vi "Eredmények FIFO-ba.vi"(8 "error in (no error)":errorcluster, 11 "Analog data":T1) -> (0 "error out":errorcluster, 3 "Analog data out":T1)   [LabVIEW 2014]
uses:
  Analog data.ctl
panel:
  out "Waveform Graph":dbl[](graph)
  out "Resistance":dbl
  out "Temperature":dbl
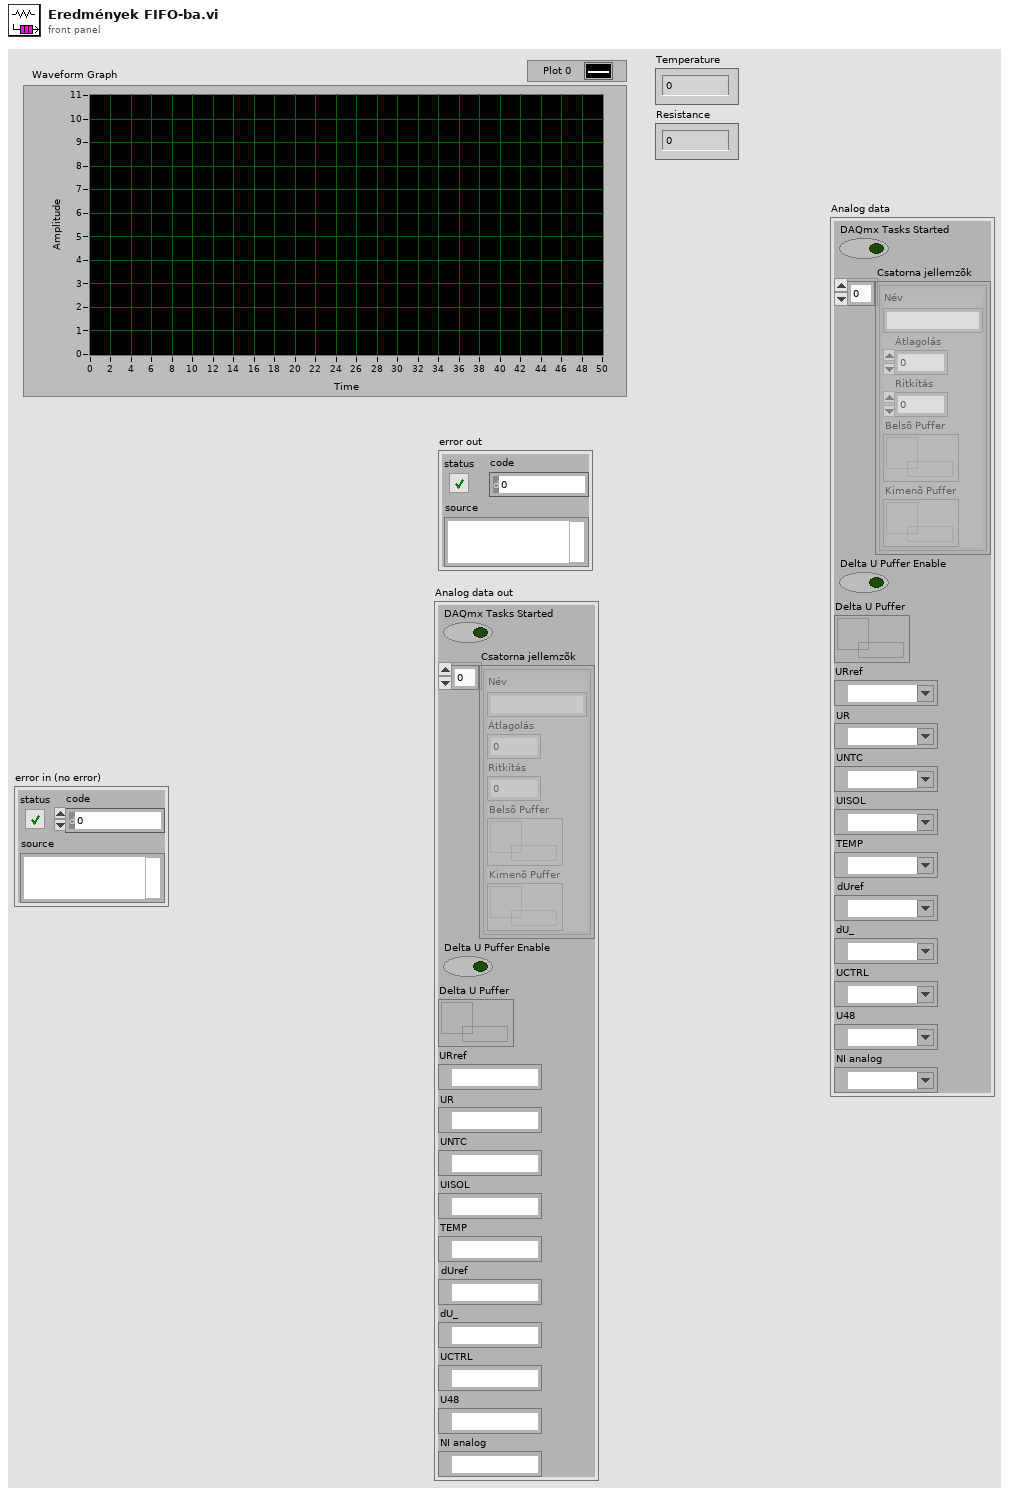
[diagram p1: front panel]
types:
  T1 = typedef "Analog data.ctl" = cluster{"DAQmx Tasks Started":bool, "Csatorna jellemzõk":T2[], "Delta U Puffer Enable":bool, "Delta U Puffer":refnum<queue>, "URref":refnum<k21>, "UR":refnum<k21>, "UNTC":refnum<k21>, "UISOL":refnum<k21>, "TEMP":refnum<k21>, "dUref":refnum<k21>, "dU_":refnum<k21>, "UCTRL":refnum<k21>, "U48":refnum<k21>, "NI analog":refnum<k21>}
  T2 = typedef "Csatorna jellemzõk.ctl" = cluster{"Név":string, "Átlagolás":i32, "Ritkítás":i32, "Belsõ Puffer":refnum<queue>, "Kimenõ Puffer":refnum<queue>}
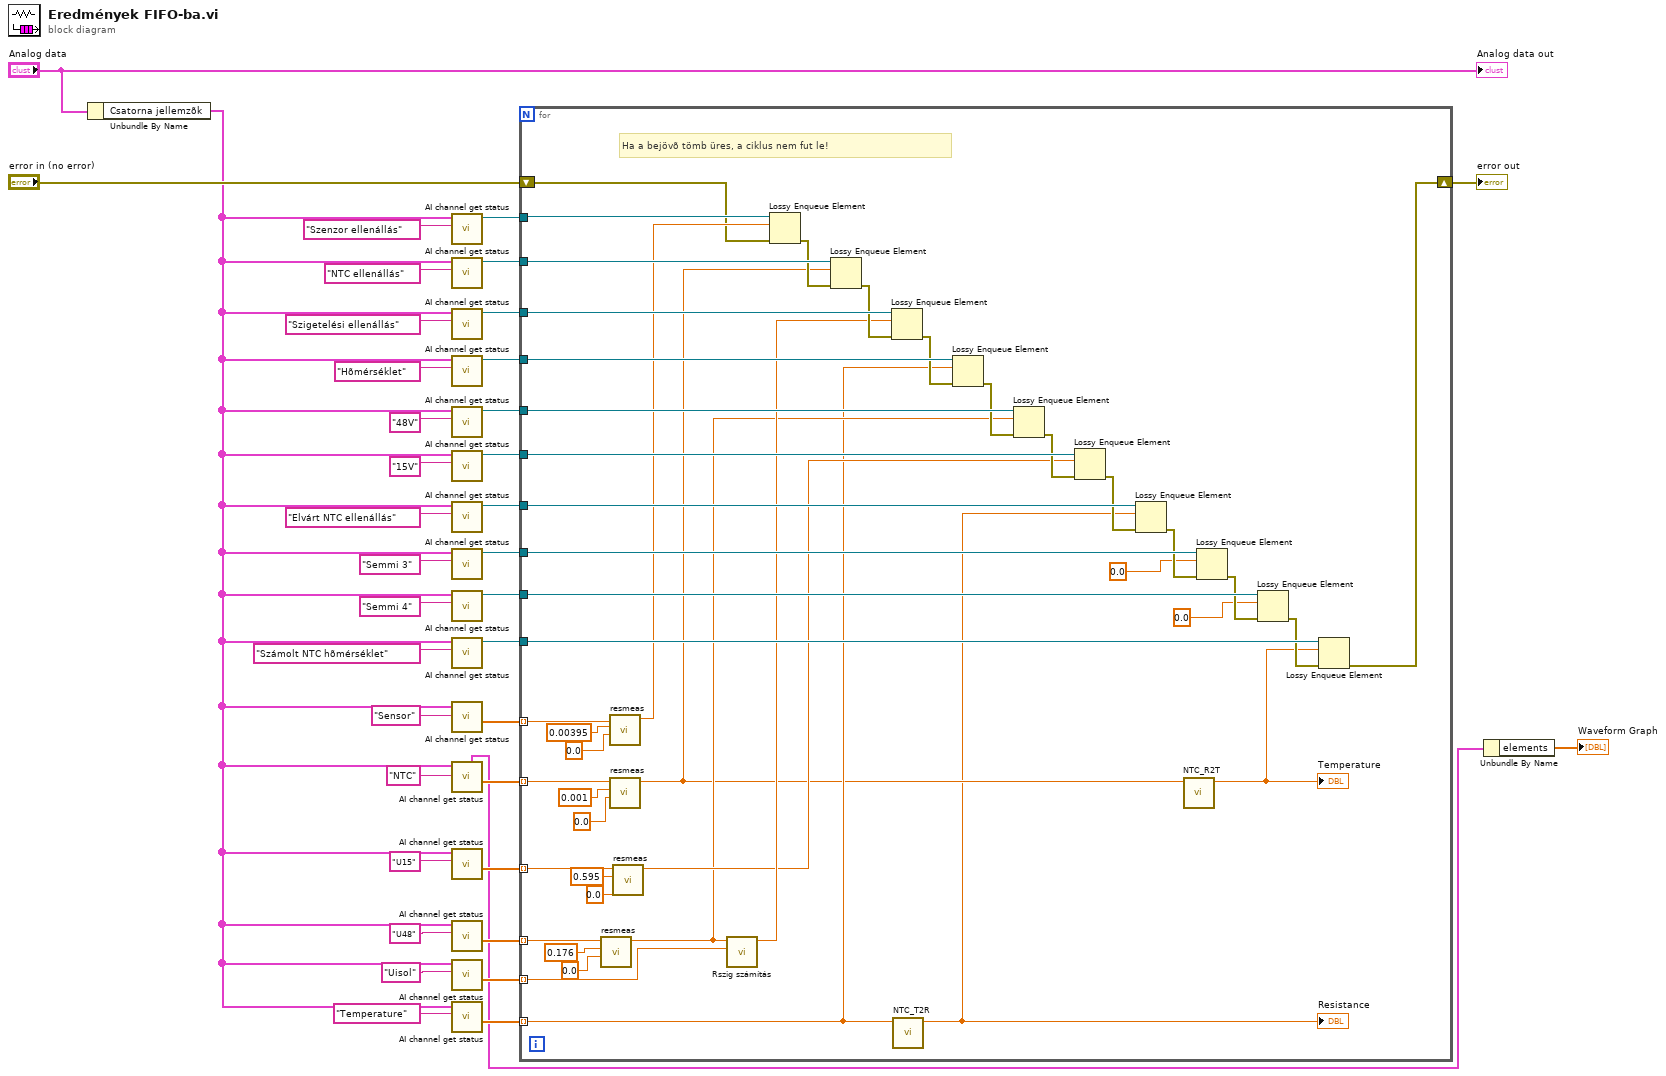
[diagram p0: block diagram]
diagram:
  n1 = Unbundle By Name("Analog data") -> ("Csatorna jellemzõk"=w4:T2[])
  n2 = call "AI channel get status.vi"("Név"="Szenzor ellenállás", "Csatorna jellemzõk"=w4) -> ("Kimenõ Puffer"=w36:refnum<queue>)  [unwired: 5 in, 4 out]
  n3 = call "AI channel get status.vi"("Név"="NTC ellenállás", "Csatorna jellemzõk"=w4) -> ("Kimenõ Puffer"=w37:refnum<queue>)  [unwired: 5 in, 4 out]
  n4 = call "AI channel get status.vi"("Név"="Szigetelési ellenállás", "Csatorna jellemzõk"=w4) -> ("Kimenõ Puffer"=w31:refnum<queue>)  [unwired: 5 in, 4 out]
  n5 = call "AI channel get status.vi"("Név"="Hõmérséklet", "Csatorna jellemzõk"=w4) -> ("Kimenõ Puffer"=w30:refnum<queue>)  [unwired: 5 in, 4 out]
  n6 = call "AI channel get status.vi"("Név"="48V", "Csatorna jellemzõk"=w4) -> ("Kimenõ Puffer"=w18:refnum<queue>)  [unwired: 5 in, 4 out]
  n7 = call "AI channel get status.vi"("Név"="15V", "Csatorna jellemzõk"=w4) -> ("Kimenõ Puffer"=w17:refnum<queue>)  [unwired: 5 in, 4 out]
  n8 = call "AI channel get status.vi"("Név"="Elvárt NTC ellenállás", "Csatorna jellemzõk"=w4) -> ("Kimenõ Puffer"=w16:refnum<queue>)  [unwired: 5 in, 4 out]
  n9 = call "AI channel get status.vi"("Név"="Semmi 3", "Csatorna jellemzõk"=w4) -> ("Kimenõ Puffer"=w15:refnum<queue>)  [unwired: 5 in, 4 out]
  n10 = call "AI channel get status.vi"("Név"="Semmi 4", "Csatorna jellemzõk"=w4) -> ("Kimenõ Puffer"=w14:refnum<queue>)  [unwired: 5 in, 4 out]
  n11 = call "AI channel get status.vi"("Név"="Számolt NTC hõmérséklet", "Csatorna jellemzõk"=w4) -> ("Kimenõ Puffer"=w13:refnum<queue>)  [unwired: 5 in, 4 out]
  n12 = call "AI channel get status.vi"("Név"="Sensor", "Csatorna jellemzõk"=w4) -> ("elements"=w12:dbl[])  [unwired: 5 in, 4 out]
  n13 = call "AI channel get status.vi"("Név"="NTC", "Csatorna jellemzõk"=w4) -> ("elements"=w7:dbl[], "Hullám"=w2:cluster{"value":dbl, dbl, "elements":dbl[]})  [unwired: 5 in, 3 out]
  n14 = call "AI channel get status.vi"("Név"="U15", "Csatorna jellemzõk"=w4) -> ("elements"=w6:dbl[])  [unwired: 5 in, 4 out]
  n15 = call "AI channel get status.vi"("Név"="U48", "Csatorna jellemzõk"=w4) -> ("elements"=w11:dbl[])  [unwired: 5 in, 4 out]
  n16 = call "AI channel get status.vi"("Név"="Uisol", "Csatorna jellemzõk"=w4) -> ("elements"=w10:dbl[])  [unwired: 5 in, 4 out]
  n17 = call "AI channel get status.vi"("Név"="Temperature", "Csatorna jellemzõk"=w4) -> ("elements"=w9:dbl[])  [unwired: 5 in, 4 out]
  n18 = for {
    tunnel: w36 -> [w82]
    tunnel: w37 -> [w81]
    shift-right: [w57] -> w3
    shift-left: "error in (no error)" -> [w41]
    tunnel: w31 -> [w79]
    tunnel: w30 -> [w78]
    tunnel: w18 -> [w75]
    tunnel: w17 -> [w73]
    tunnel: w16 -> [w71]
    tunnel: w15 -> [w69]
    tunnel: w14 -> [w68]
    tunnel: w13 -> [w67]
    tunnel: w12 -> [w42] mode=indexing
    tunnel: w11 -> [w49] mode=indexing
    tunnel: w10 -> [w56] mode=indexing
    tunnel: w9 -> [w44] mode=indexing
    tunnel: w7 -> [w58] mode=indexing
    tunnel: w6 -> [w53] mode=indexing
    # "Ha a bejövõ tömb üres, a ciklus nem fut le!"
    n19 = call "resmeas.vi"("Rc"=0.0, "Im"=0.176, "Um"=w49) -> ("Rm"=w46:dbl)  [unwired: 8 in]
    n20 = call "resmeas.vi"("Rc"=0.0, "Im"=0.00395, "Um"=w42) -> ("Rm"=w45:dbl)  [unwired: 8 in]
    n21 = call "resmeas.vi"("Rc"=0.0, "Im"=0.001, "Um"=w58) -> ("Rm"=w43:dbl)  [unwired: 8 in]
    n22 = call "resmeas.vi"("Rc"=0.0, "Im"=0.595, "Um"=w53) -> ("Rm"=w50:dbl)  [unwired: 8 in]
    n23 = call "Rszig számítás.vi"("UIsol"=w56, "U48"=w46) -> ("Rszig"=w59:dbl)  [unwired: 9 in]
    n24 = Lossy Enqueue Element(queue=w82, element=w45, error in (no error)=w41) -> (error out=w80:errorcluster)  [unwired: 3 out]
    n25 = Lossy Enqueue Element(queue=w81, element=w43, error in (no error)=w80) -> (error out=w77:errorcluster)  [unwired: 3 out]
    n26 = Lossy Enqueue Element(queue=w79, element=w59, error in (no error)=w77) -> (error out=w76:errorcluster)  [unwired: 3 out]
    n27 = call "NTC_T2R.vi"("Temperature"=w44) -> ("Resistance"=w40:dbl)  [unwired: 10 in]
    "Resistance" <- w40
    n28 = Lossy Enqueue Element(queue=w78, element=w44, error in (no error)=w76) -> (error out=w74:errorcluster)  [unwired: 3 out]
    n29 = Lossy Enqueue Element(queue=w75, element=w46, error in (no error)=w74) -> (error out=w72:errorcluster)  [unwired: 3 out]
    n30 = Lossy Enqueue Element(queue=w73, element=w50, error in (no error)=w72) -> (error out=w70:errorcluster)  [unwired: 3 out]
    n31 = Lossy Enqueue Element(queue=w71, element=w40, error in (no error)=w70) -> (error out=w66:errorcluster)  [unwired: 3 out]
    n32 = call "NTC_R2T.vi"("Resistance"=w43) -> ("Temperature"=w39:dbl)  [unwired: 10 in]
    "Temperature" <- w39
    n33 = Lossy Enqueue Element(queue=w69, element=0.0, error in (no error)=w66) -> (error out=w65:errorcluster)  [unwired: 3 out]
    n34 = Lossy Enqueue Element(queue=w68, element=0.0, error in (no error)=w65) -> (error out=w64:errorcluster)  [unwired: 3 out]
    n35 = Lossy Enqueue Element(queue=w67, element=w39, error in (no error)=w64) -> (error out=w57:errorcluster)  [unwired: 3 out]
  }
  "error out" <- w3
  n36 = Unbundle By Name(w2) -> ("elements"=→"Waveform Graph":dbl[])
  "Analog data out" <- "Analog data"
